vi "slscswitch Reset.vi"(8 "error in (no error)":errorcluster, 11 "SLSC Switch in":refnum<class "SLSC Switch.lvclass">) -> (0 "error out":errorcluster, 3 "SLSC Switch out":refnum<class "SLSC Switch.lvclass">)   [LabVIEW 2015, in "SLSC Switch.lvclass"]
uses:
  SLSC Switch.lvclass
  SLSC Switch.lvclass/SLSC Switch.ctl
  <vilib>/SLSC/SLSC.lvlib
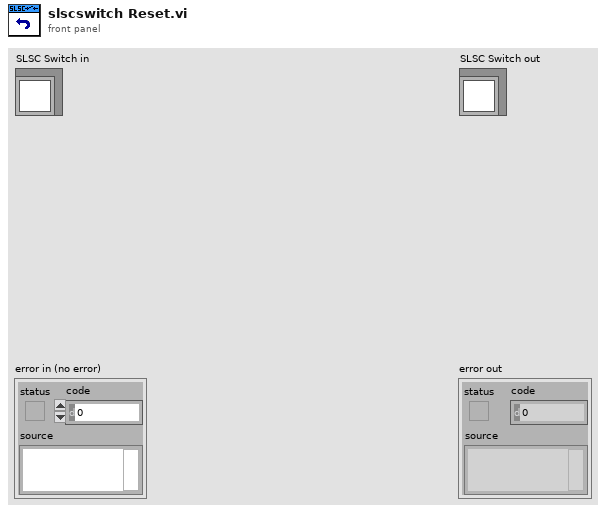
[diagram p1: front panel]
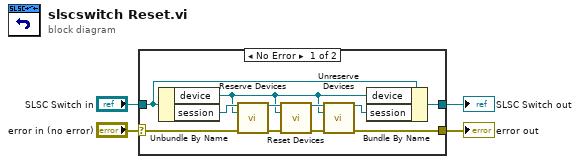
[diagram p0: block diagram]
diagram:
  n1 = case shown="No Error" "error in (no error)" {
    selector: "error in (no error)" -> [w6 w17]
    tunnel: [w5 w17] -> w3
    tunnel: [w11 w16] -> w1
    tunnel: "SLSC Switch in" -> [w10 w16]
    frame No Error {
      n2 = Unbundle By Name(w10) -> ("device"=w8:refnum<k21>, "session"=w9:refnum<k21>)
      n3 = call <vilib>:"Reserve Devices.vi"("session in"=w9, "devices"=w8, "error in (no error)"=w6) -> ("session out"=w15:refnum<k21>, "error out"=w14:errorcluster)  [unwired: 11 in]
      n4 = call <vilib>:"Reset Devices.vi"("session in"=w15, "devices"=w8, "error in (no error)"=w14) -> ("session out"=w13:refnum<k21>, "error out"=w12:errorcluster)  [unwired: 11 in]
      n5 = call <vilib>:"Unreserve Devices.vi"("session in"=w13, "devices"=w8, "error in (no error)"=w12) -> ("session out"=w7:refnum<k21>, "error out"=w5:errorcluster)  [unwired: 11 in]
      n6 = Bundle By Name(cluster=w10, "device"=w8, "session"=w7) -> (w11:refnum<class "SLSC Switch.lvclass">)
    }
    frame Error {
    }
  }
  "error out" <- w3
  "SLSC Switch out" <- w1
